vi "Create Buffers.vi"(8 "error in (no error)":errorcluster, 11 "Historian Module in":refnum<class "Historian Module.lvclass">) -> (0 "error out":errorcluster, 3 "Historian Module out":refnum<class "Historian Module.lvclass">)   [LabVIEW 2020, in "VolatusHistorian.lvlib" / "Historian Module.lvclass"]
uses:
  Historian Module.lvclass
  C:/dev/lv20CE/relink/lv-volatus/Volatus/Module/Module.lvclass
  Volatus/Module/Module.lvclass/Module.ctl
  Historian Module.lvclass/Historian Module.ctl
  VolatusConfig/VolatusConfigElement/VolatusConfigElement.lvclass/VolatusConfigElement.ctl
  Volatus/Module/Config.vi
  VolatusConfig/VolatusConfigElement/Element.vi
  VolatusConfig/Group/Group Config.lvclass
  C:/dev/lv20CE/relink/lv-volatus/VolatusConfig/VolatusConfigElement/VolatusConfigElement.lvclass
  VolatusConfig/Channel/Channel Config.lvclass
  Group Data Handler/Group Data Handler.lvclass
  C:/dev/lv20CE/relink/lv-vecto/Vecto/SubscribedDataHandler/SubscribedDataHandler.lvclass
  VolatusConfig/Task/Task Config.lvclass
  Group Buffer DBL/Group Buffer DBL.lvclass
  Volatus/Module/Module.lvclass
  VolatusConfig/Cluster/Cluster Config.lvclass
  VolatusConfig/VolatusConfig.lvlib
  VolatusConfig/VolatusConfigElement/VolatusConfigElement.lvclass
  Volatus/VolatusAPI/VolatusAPI.lvclass
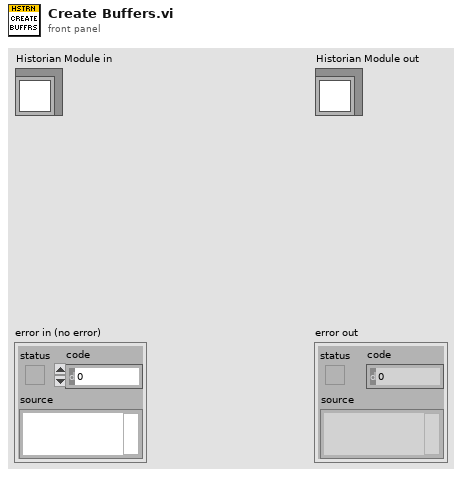
[diagram p1: front panel]
types:
  T1 = map{string, refnum<class "Group Buffer DBL.lvclass">}
  T2 = typedef "VectoConfig.lvlib/Group Data Type.ctl" = enum16{"Double", "String", "Bool"}
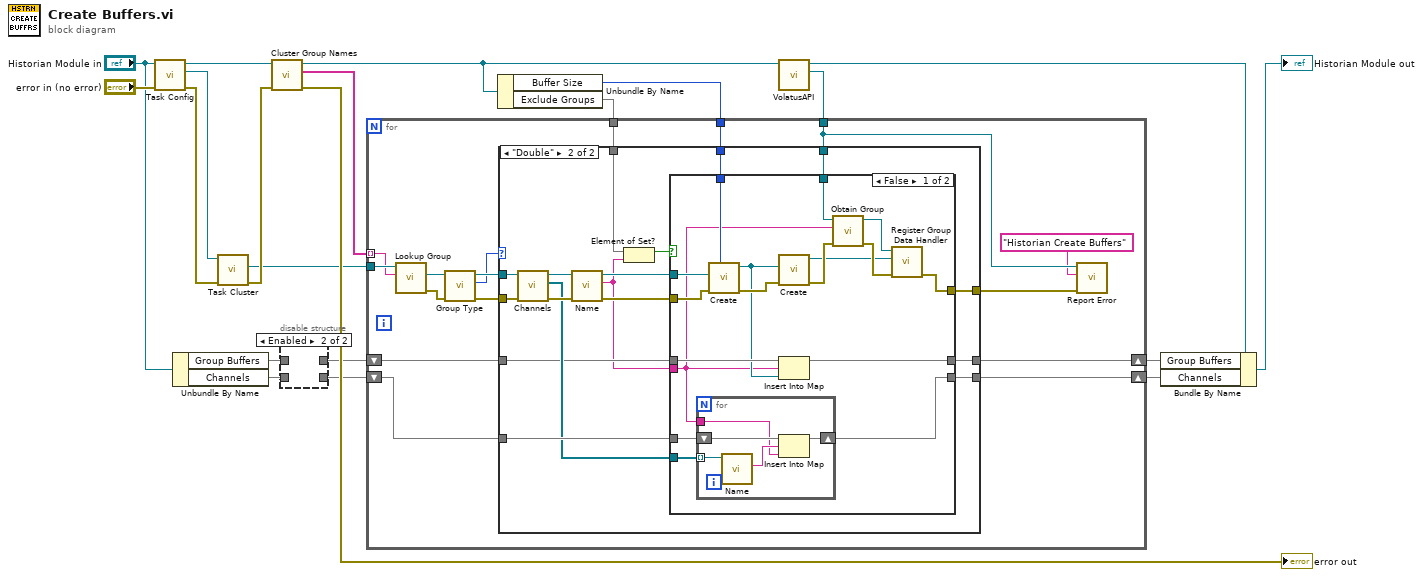
[diagram p0: block diagram]
diagram:
  n1 = call "Task Config.vi"("error in (no error)"="error in (no error)", "Module in"="Historian Module in") -> ("error out"=w15:errorcluster, "Task Config"=w17:refnum<class "Task Config.lvclass">, "Module out"=w18:refnum<class "Historian Module.lvclass">)  [unwired: 7 in]
  n2 = Unbundle By Name("Historian Module in") -> ("Group Buffers"=w9:T1, "Channels"=w7:map{string, string})
  n3 = call "Task Cluster.vi"("error in (no error)"=w15, "Task Config in"=w17) -> ("error out"=w20:errorcluster, "Cluster"=w16:refnum<class "Cluster Config.lvclass">)  [unwired: 7 in, 1 out]
  n4 = call "Cluster Group Names.vi"("error in (no error)"=w20, "Historian Module in"=w18) -> ("error out"=→"error out":errorcluster, "Group Names"=w14:string[], "Historian Module out"=w13:refnum<class "Historian Module.lvclass">)  [unwired: 7 in]
  n5 = disable-structure shown="Enabled" {
    disable-tunnel: [w23 _] -> w10
    disable-tunnel: w9 -> [w23 _]
    disable-tunnel: [w22 _] -> w8
    disable-tunnel: w7 -> [w22 _]
    frame Disabled {
    }
    frame Enabled {
    }
  }
  n6 = Unbundle By Name(w13) -> ("Buffer Size"=w12:i32, "Exclude Groups"=w3:set{string})
  n7 = call "VolatusAPI.vi"("Module in"=w13) -> ("VolatusAPI"=w1:refnum<class "VolatusAPI.lvclass">, "Module out"=w2:refnum<class "Historian Module.lvclass">)  [unwired: 9 in]
  n8 = for {
    tunnel: w16 -> [w39]
    tunnel: w14 -> [w38] mode=indexing
    tunnel: w12 -> [w37]
    shift-right: [w33] -> w5
    shift-left: w10 -> [w34]
    shift-right: [w35] -> w4
    shift-left: w8 -> [w36]
    tunnel: w3 -> [w32]
    tunnel: w1 -> [w25]
    n9 = call "Lookup Group.vi"("Group Name"=w38, "Cluster in"=w39) -> ("error out"=w30:errorcluster, "Group"=w31:refnum<class "Group Config.lvclass">)  [unwired: 6 in, 2 out]
    n10 = call "Group Type.vi"("error in (no error)"=w30, "Group in"=w31) -> ("error out"=w29:errorcluster, "Group Data Type"=w27:T2, "Group out"=w28:refnum<class "Group Config.lvclass">)  [unwired: 7 in]
    n11 = case shown="\"Double\"" w27 {
      tunnel: w37 -> [_ w59]
      tunnel: [w42 w54] -> w26
      tunnel: w36 -> [w40 w53]
      tunnel: [w40 w51] -> w35
      tunnel: w34 -> [w41 w50]
      tunnel: [w41 w49] -> w33
      tunnel: w32 -> [_ w47]
      tunnel: w25 -> [_ w45]
      tunnel: w29 -> [w42 w44]
      tunnel: w28 -> [_ w43]
      frame "String", "Bool" {
        # "Only Double supported for now."
      }
      frame "Double" {
        n12 = call "Channels.vi"("error in (no error)"=w44, "Group in"=w43) -> ("error out"=w57:errorcluster, "Channels"=w52:refnum<class "Channel Config.lvclass">[], "Group out"=w58:refnum<class "Group Config.lvclass">)  [unwired: 7 in]
        n13 = call "Name.vi"("error in (no error)"=w57, "VolatusConfigElement in"=w58) -> ("error out"=w56:errorcluster, "Name"=w48:string, "VolatusConfigElement out"=w55:refnum<class "Group Config.lvclass">)  [unwired: 7 in]
        n14 = Element of Set?(10:w48, 11:w47) -> (3:w46:bool)
        n15 = case shown="False" w46 {
          tunnel: w59 -> [w73 _]
          tunnel: w56 -> [w72 w84]
          tunnel: w55 -> [w71 _]
          tunnel: [w63 w84] -> w54
          tunnel: w53 -> [w70 w82]
          tunnel: w52 -> [w69 _]
          tunnel: [w68 w82] -> w51
          tunnel: w50 -> [w67 w83]
          tunnel: [w66 w83] -> w49
          tunnel: w48 -> [w62 _]
          tunnel: w45 -> [w61 _]
          frame False {
            n16 = for {
              shift-right: [w77] -> w68
              shift-left: w70 -> [w80]
              tunnel: w62 -> [w78]
              tunnel: w69 -> [w81] mode=indexing
              n17 = call "Name.vi"("VolatusConfigElement in"=w81) -> ("Name"=w79:string)  [unwired: 8 in, 2 out]
              n18 = Insert Into Map(map in=w80, key=w79, value=w78) -> (map out=w77:map{string, string})  [unwired: 2 out]
            }
            n19 = call "Create.vi"("Size"=w73, "error in (no error)"=w72, "Group Config"=w71) -> ("error out"=w74:errorcluster, "Group Buffer DBL out"=w65:refnum<class "Group Buffer DBL.lvclass">)  [unwired: 7 in]
            n20 = call "Create.vi"("error in (no error)"=w74, "Group Buffer"=w65) -> ("error out"=w75:errorcluster, "Group Data Handler out"=w64:refnum<class "Group Data Handler.lvclass">)  [unwired: 8 in]
            n21 = Insert Into Map(map in=w67, key=w62, value=w65) -> (map out=w66:T1)  [unwired: 2 out]
            n22 = call "Obtain Group.vi"("error in (no error)"=w75, "Group Name"=w62, "VolatusAPI in"=w61) -> ("error out"=w76:errorcluster, "VolatusAPI out"=w60:refnum<class "VolatusAPI.lvclass">)  [unwired: 6 in, 1 out]
            n23 = call "Register Group Data Handler.vi"("error in (no error)"=w76, "Data Handler"=w64, "VolatusAPI in"=w60) -> ("error out"=w63:errorcluster)  [unwired: 7 in, 1 out]
          }
          frame True {
          }
        }
      }
    }
    n24 = call "Report Error.vi"("error in (no error)"=w26, "Context"="Historian Create Buffers", "VolatusAPI in"=w25) -> ()  [unwired: 7 in, 2 out]
  }
  n25 = Bundle By Name(cluster=w2, "Group Buffers"=w5, "Channels"=w4) -> (→"Historian Module out":refnum<class "Historian Module.lvclass">)
